vi "FT_Get_Device_Info_64bit.vi"(8 "error in (no error)":errorcluster, 11 "Handle":u64) -> (0 "error out":errorcluster, 1 "Device Information":T1 {"Type" items=["FT232B-FT245B", "FT8U232AM-FT8U245AM", "FT8U100AX", "UNKNOWN", "FT2232", "FT232R-FT245R", "FT2232H", "FT4232H", "FT232H"]}, 2 "FT_Status":u32(ring) items=["FT_OK", "FT_INVALID_HANDLE", "FT_DEVICE_NOT_FOUND", "FT_DEVICE_NOT_OPENED", "FT_IO_ERROR", "FT_INSUFFICIENT_RESOURCES", "FT_INVALID_PARAMETER", "FT_INVALID_BAUD_RATE", "FT_DEVICE_NOT_OPENED_FOR_ERASE", "FT_DEVICE_NOT_OPENED_FOR_WRITE", "FT_FAILED_TO_WRITE_DEVICE", "FT_EEPROM_READ_FAILED", "FT_EEPROM_WRITE_FAILED", "FT_EEPROM_ERASE_FAILED", "FT_EEPROM_NOT_PRESENT", "FT_EEPROM_NOT_PROGRAMMED", "FT_INVALID_ARGS", "FT_NOT_SUPPORTED", "FT_OTHER_ERROR"], 3 "Handle out":u64)   [LabVIEW 2019]
uses:
  FTD2XX.dll
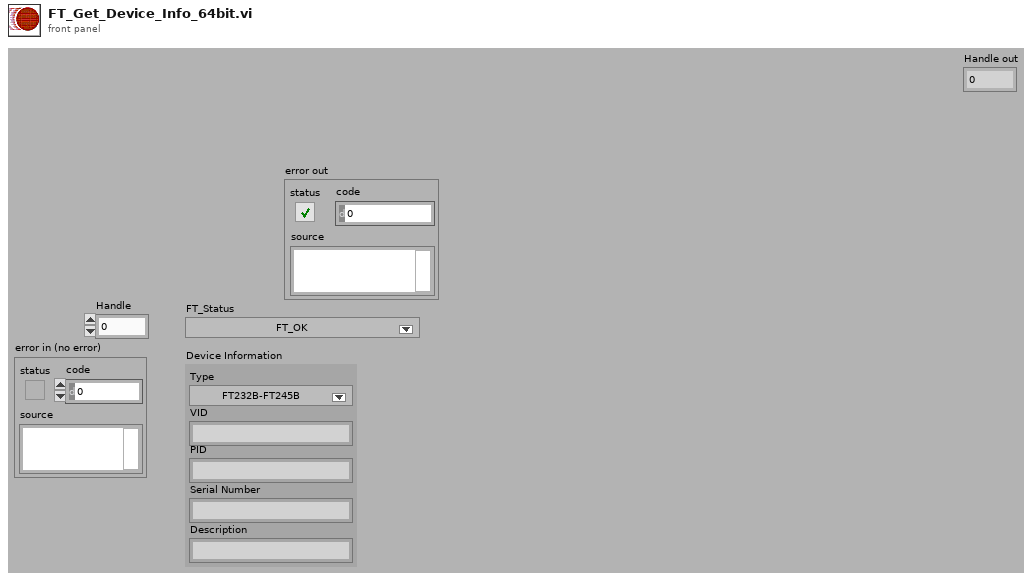
[diagram p1: front panel]
types:
  T1 = cluster{"Type":u32, "VID":string, "PID":string, "Serial Number":string, "Description":string}
  T2 = cluster{"DeviceType":u32, string, string, "SerialNumber":string, "Description":string}
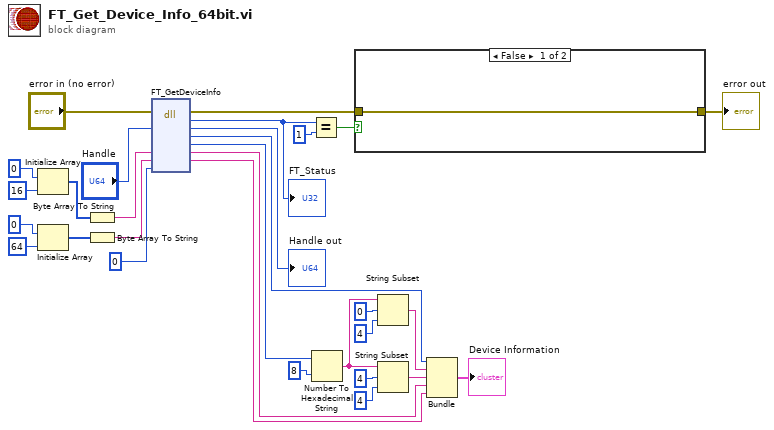
[diagram p0: block diagram]
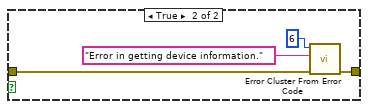
[diagram p2: hidden frame]
diagram:
  n1 = Initialize Array(u8 0, 16 ("dimension size")) -> (w15:u8[])
  n2 = Initialize Array(u8 0, 64 ("dimension size")) -> (w13:u8[])
  n3 = Byte Array To String(unsigned byte array=w15) -> (string=w9:string)
  n4 = Byte Array To String(unsigned byte array=w13) -> (string=w10:string)
  n5 = dll-call lib="FTD2XX.dll" fn="FT_GetDeviceInfo"(error in="error in (no error)", "Handle"="Handle", "SerialNumber"=w9, "Description"=w10, "Dummy"=u32 0) -> (error out=w3:errorcluster, "FT_Status"=w4:u32, "Handle"=→"Handle out":u64, "DeviceType"=w8:u32, "ID"=w29:u32, "SerialNumber"=w20:string, "Description"=w19:string)  [unwired: 5 in, 1 out]
  "FT_Status" <- w4
  n6 = Equal?(x=w4, y=u32 1) -> (x = y?=w6:bool)
  n7 = Number To Hexadecimal String(1:i16 8 ("width (-)"), 2:w29) -> (0:w23:string)
  n8 = case shown="False" w6 {
    tunnel: [w31 w34] -> w7
    tunnel: w3 -> [w31 w33]
    frame False {
    }
    frame True {
      n9 = call <vilib>:"Error Cluster From Error Code.vi"("error in (no error)"=w33, "error message (\"\")"="Error in getting device information." ("error message (\"\")"), "error code (0)"=6) -> ("error out"=w34:errorcluster)  [unwired: 6 in]
    }
  }
  "error out" <- w7
  n10 = String Subset(string=w23, offset (0)=0, length (rest)=4 ("length (rest)")) -> (substring=w22:string)
  n11 = String Subset(string=w23, offset (0)=4, length (rest)=4 ("length (rest)")) -> (substring=w21:string)
  n12 = Bundle("DeviceType"=w8, w22, w21, "SerialNumber"=w20, "Description"=w19) -> (→"Device Information":T2)  [unwired: 1 in]
